vi "testing02.vi"() -> ()   [LabVIEW 2017]
panel:
  in  "Set DAC":bool
  in  "DAC, V":dbl min=-10.0 max=10.0
  in  "Exit":bool
  in  "COM port":refnum<visa-resource-name>
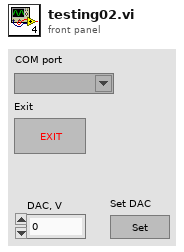
[diagram p1: front panel]
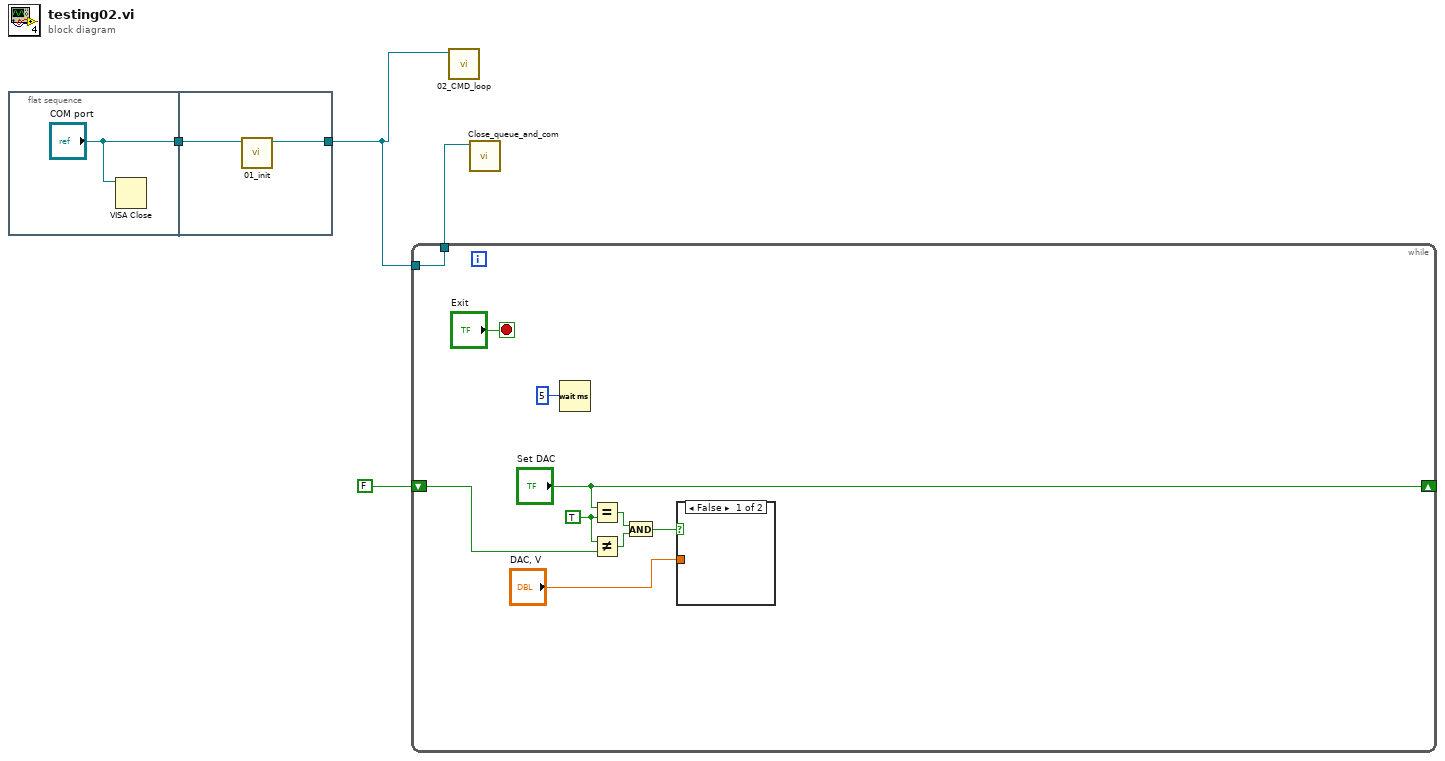
[diagram p0: block diagram]
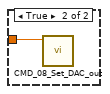
[diagram p2: hidden frame]
diagram:
  n1 = flat-sequence {
    tunnel: ["COM port"] -> w4
    tunnel: w4 -> [w7]
    tunnel: [w6] -> w1
    frame #0 {
      n2 = VISA Close(VISA resource name="COM port") -> ()  [unwired: 1 in, 1 out]
    }
    frame #1 {
      n3 = call "01_init.vi"("COM port"=w7) -> ("VISA resource name out"=w6:refnum<visa-resource-name>)  [unwired: 8 in, 2 out]
    }
  }
  n4 = while {
    tunnel: w1 -> [w16]
    tunnel: [w16] -> w3
    shift-right: ["Set DAC"] -> _
    shift-left: FALSE ("Set Waveform") -> [w10]
    stop <- "Exit" stop-if-true
    w15 = TRUE ("y")
    n5 = Wait (ms)(milliseconds to wait=u32 5) -> ()  [unwired: 1 out]
    n6 = Equal?(x="Set DAC", y=w15) -> (x = y?=w14:bool)
    n7 = Not Equal?(x=w15, y=w10) -> (x != y?=w13:bool)
    n8 = And(x=w14, y=w13) -> (x .and. y?=w12:bool)
    n9 = case shown="False" w12 {
      tunnel: "DAC, V" -> [_ w18]
      frame False {
      }
      frame True {
        n10 = call "CMD_08_Set_DAC_out.vi"("DAC voltage, V"=w18) -> ()  [unwired: 11 in]
      }
    }
  }
  n11 = call "02_CMD_loop.vi"("VISA resource name"=w1) -> ()  [unwired: 11 in]
  n12 = call "Close_queue_and_com.vi"("VISA"=w3) -> ()  [unwired: 11 in]
